vi "Number Payloads Available.vi"(8 "error in (no error)":errorcluster, 11 "Basic WebSocket Manager in":refnum<class "Basic WebSocket Manager.lvclass">) -> (0 "error out":errorcluster, 2 "# Payloads":i32, 3 "Basic WebSocket Manager out":refnum<class "Basic WebSocket Manager.lvclass">)   [LabVIEW 2020, in "HTTP Server.lvlib" / "Basic WebSocket Manager.lvclass"]
uses:
  Basic WebSocket Manager.lvclass
  Basic WebSocket Manager.lvclass/Basic WebSocket Manager.ctl
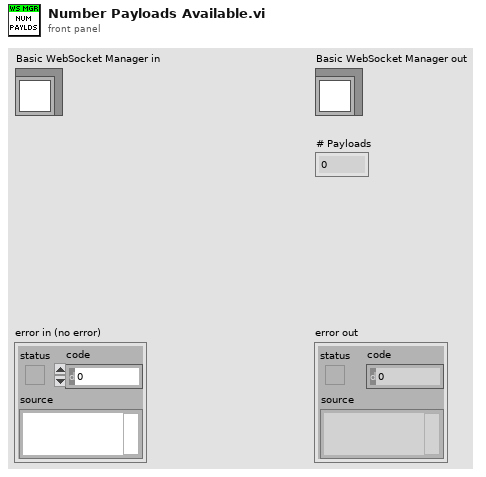
[diagram p1: front panel]
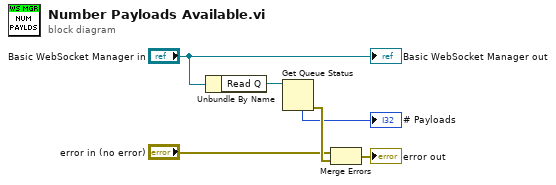
[diagram p0: block diagram]
diagram:
  n1 = Unbundle By Name("Basic WebSocket Manager in") -> ("Read Q"=w3:refnum<queue>)
  n2 = Get Queue Status(queue=w3) -> (error out=w6:errorcluster, # elements in queue=→"# Payloads":i32)  [unwired: 2 in, 6 out]
  n3 = Merge Errors("error in (no error)", w6) -> (→"error out":errorcluster)
  "Basic WebSocket Manager out" <- "Basic WebSocket Manager in"
